vi "Divide.vi"() -> ()   [LabVIEW 2025]
panel:
  out "Numeric":dbl
  out "Boolean":bool
  in  "Numeric 2":dbl
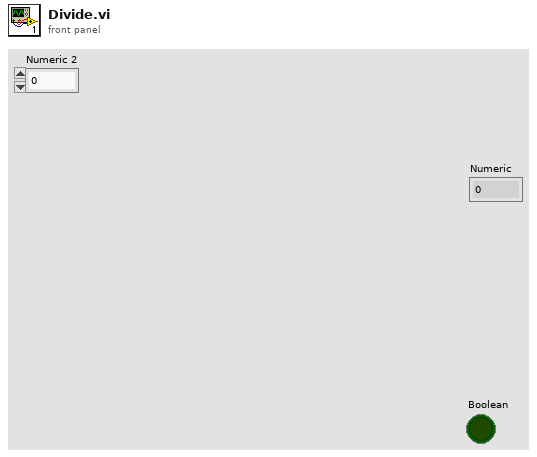
[diagram p1: front panel]
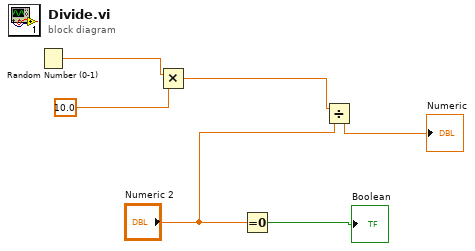
[diagram p0: block diagram]
diagram:
  n1 = Random Number (0-1) ("Random Number (0.0-10.0)")() -> (number: 0 to 1=w6:dbl)
  n2 = Multiply(x=w6, y=10.0) -> (x*y=w4:dbl)
  n3 = Equal To 0?(x="Numeric 2") -> (x = 0?=→"Boolean":bool)
  n4 = Divide(x=w4, y="Numeric 2") -> (x/y=→"Numeric":dbl)
